vi "Protocol.RQST Wait on Response.vi"(0 "ref in":T3, 1 "Ignore Response":bool, 2 "Name":string, 5 "Source Address":u8=27, 7 "PGN":u32, 9 "DA":u8, 11 "error in (no error)":errorcluster, 12 "Processed Outgoing":refnum<queue>) -> (4 "element":T1 {"payload" format="%x"; "timestamp" format="%<%.7X\n%x>T"; "type" items=["CAN Data"=0, "CAN Remote"=1, "CAN Bus Error"=2, "CAN 2.0 Data"=8, "CAN FD Data"=16, "CAN FD+BRS Data"=24, "J1939 Data"=192, "Delay"=224, "Log Trigger"=225, "Start Trigger"=226]; "identifier" format="%x"}, 6 "timed out?":bool, 8 "Global Request?":bool, 15 "error out":errorcluster)   [LabVIEW 2019, in "J1939 Addon Engine.lvlib"]
uses:
  J1939 Addon Engine.lvlib
  Types/Protocol.RQST Lookup Table Reference.ctl
  <vilib>/xnet/xnet.llb/XNET Frame CAN.ctl
  <vilib>/xnet/xnet.llb/XNET Frame Type CAN.ctl
  Support Libraries/J1939 Utilities/Types/CAN Outgoing Message Cluster.ctl
  Types/Protocol.RQST Lookup Table Action.ctl
  Types/Protocol.RQST Lookup Table Cluster.ctl
  Support Libraries/J1939 Utilities/SubVIs/Request.vi
  Support Libraries/J1939 Utilities/Common Conversions.vi
  Support Libraries/J1939 Utilities/SubVIs/Convert J1939 ID to CAN Arb ID.vi
  Protocol.RQST Lookup Table.vi
  Support Libraries/J1939 Utilities/J1939 Utilities.lvlib
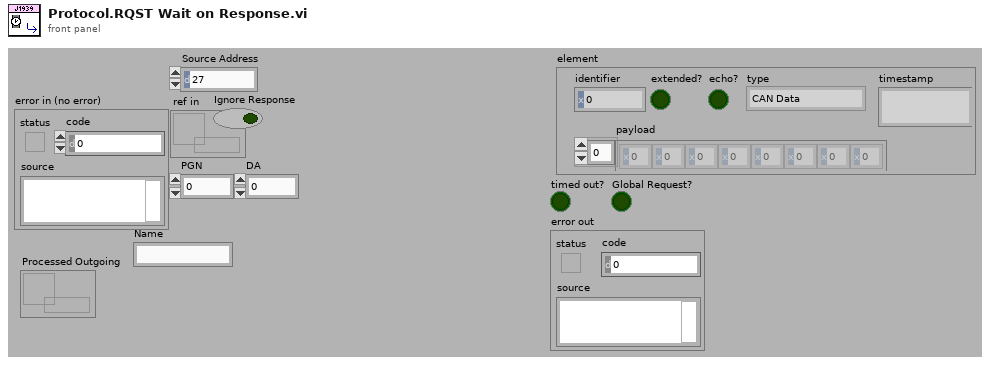
[diagram p1: front panel]
types:
  T1 = typedef "XNET Frame CAN.ctl" = cluster{"timestamp":timestamp, "payload":u8[], "identifier":u32, "type":T2, "extended?":bool, "echo?":bool}
  T2 = typedef "XNET Frame Type CAN.ctl" = u8
  T3 = typedef "J1939 Addon Engine.lvlib/Protocol.RQST Lookup Table Reference.ctl" = refnum<data-value>
  T4 = typedef "J1939 Utilities.lvlib/CAN Outgoing Message Cluster.ctl" = cluster{"Identifier":u32, "Data":u8[]}
  T5 = typedef "J1939 Addon Engine.lvlib/Protocol.RQST Lookup Table Action.ctl" = enum16{"Initialize", "Add", "Get", "Remove", "Get Active Requests"}
  T6 = typedef "J1939 Addon Engine.lvlib/Protocol.RQST Lookup Table Cluster.ctl" = cluster{"Response Q":refnum<queue>, "Request PGN":u32}
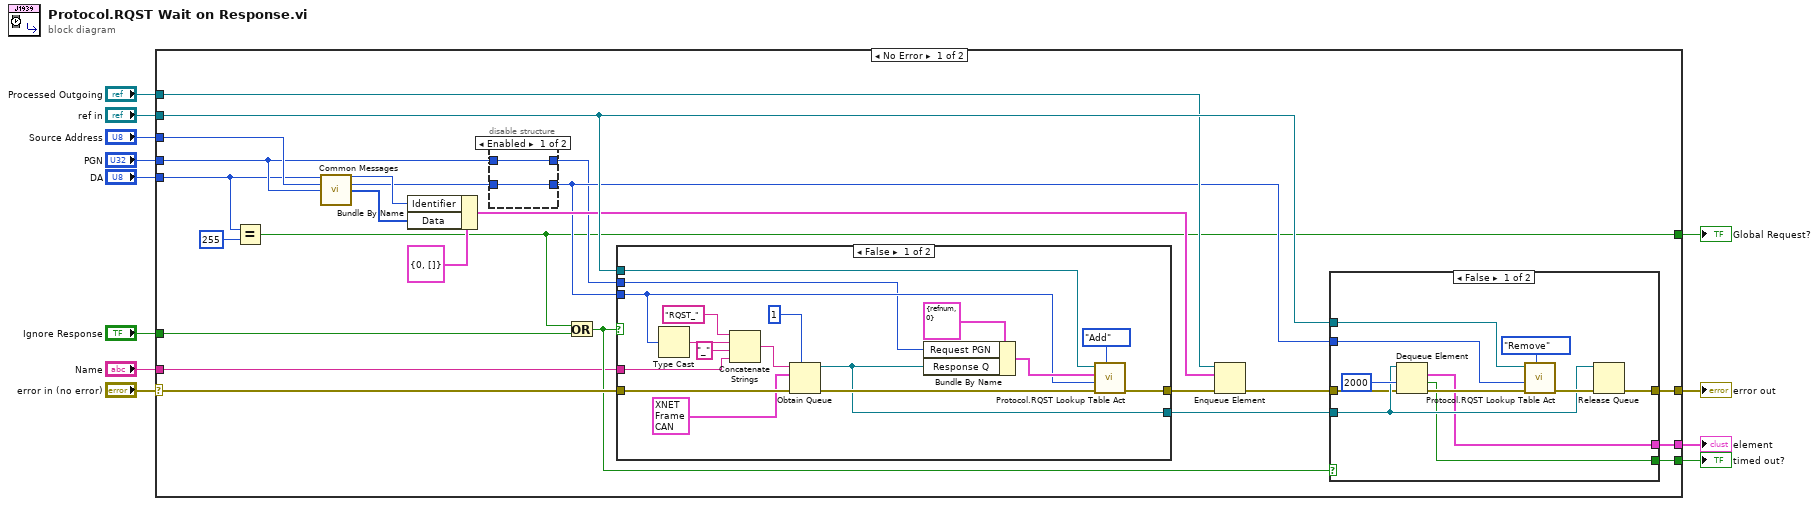
[diagram p0: block diagram]
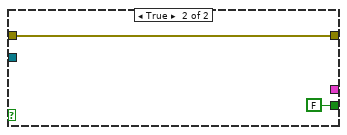
[diagram p2: hidden frame]
diagram:
  n1 = case shown="No Error" "error in (no error)" {
    selector: "error in (no error)" -> [w36 w71]
    tunnel: "Source Address" -> [w20 _]
    tunnel: "ref in" -> [w35 _]
    tunnel: [w33 w71] -> w8
    tunnel: [w32 _] -> w10
    tunnel: [w31 _] -> w9
    tunnel: "Processed Outgoing" -> [w28 _]
    tunnel: "PGN" -> [w19 _]
    tunnel: "DA" -> [w18 _]
    tunnel: [w14 _] -> w3
    tunnel: "Ignore Response" -> [w16 _]
    tunnel: "Name" -> [w13 _]
    frame No Error {
      n2 = Equal?(x=w18, y=u8 255) -> (x = y?=w14:bool)
      n3 = call-poly "Common Messages.vi"("Destination Address"=w18, "Source Address"=w20, "PGN"=w19) -> ("Arb ID"=w25:u32, "Expected Return Arb ID"=w23:u32, "Data"=w26:u8[])  [unwired: 10 in]
      n4 = Bundle By Name(cluster=T4 {"Identifier"=0, "Data"=[]} ("element"), "Identifier"=w25, "Data"=w26) -> (w24:T4)
      n5 = disable-structure shown="Enabled" {
        disable-tunnel: [w69 w70] -> w22
        disable-tunnel: w23 -> [w69 _]
        disable-tunnel: w19 -> [w68 w70]
        disable-tunnel: [w68 w70] -> w21
        frame Enabled {
        }
        frame Disabled {
        }
      }
      n6 = Or(x=w14, y=w16) -> (x .or. y?=w15:bool)
      n7 = case shown="False" w15 {
        tunnel: w36 -> [w65 w67]
        tunnel: w35 -> [w60 _]
        tunnel: [w59 _] -> w34
        tunnel: [w58 w67] -> w30
        tunnel: w22 -> [w52 _]
        tunnel: w21 -> [w51 _]
        tunnel: w13 -> [w53 _]
        frame False {
          n8 = Type Cast(x=w52) -> (*(type *) &x=w57:string)  [unwired: 1 in]
          n9 = Concatenate Strings("RQST_" ("string"), w57, "_" ("string"), w53) -> (w56:string)
          n10 = Obtain Queue(max queue size (-1, unlimited)=1, name (unnamed)=w56, element data type=T1 {"timestamp"=timestamp(0 s since 1904-01-01), "payload"=[], "identifier"=0, "type"=0, "extended?"=FALSE, "echo?"=FALSE} ("CAN frame"), error in (no error)=w65) -> (queue out=w59:refnum<queue>, error out=w64:errorcluster)  [unwired: 1 in, 1 out]
          n11 = Bundle By Name(cluster=T6 {"Response Q"=refnum, "Request PGN"=0} ("Data"), "Request PGN"=w51, "Response Q"=w59) -> (w61:T6)
          n12 = call "Protocol.RQST Lookup Table Act.vi"("Action"=Protocol.RQST_Lookup_Table_Action."Add", "error in (no error)"=w64, "ID"=w52, "Data"=w61, "Rqst LUT"=w60) -> ("error out"=w58:errorcluster)  [unwired: 2 in, 4 out]
        }
        frame True {
        }
      }
      n13 = Enqueue Element(queue=w28, element=w24, error in (no error)=w30) -> (error out=w29:errorcluster)  [unwired: 1 in, 2 out]
      n14 = case shown="False" w15 {
        tunnel: w35 -> [w45 _]
        tunnel: w34 -> [w43 _]
        tunnel: [w42 w49] -> w33
        tunnel: [w41 _] -> w32
        tunnel: [w40 FALSE ("timed out?")] -> w31
        tunnel: w29 -> [w39 w49]
        tunnel: w22 -> [w38 _]
        frame False {
          n15 = Dequeue Element(queue=w43, timeout in ms (-1)=2000, error in (no error)=w39) -> (element=w41:T1, timed out?=w40:bool, error out=w46:errorcluster)  [unwired: 1 out]
          n16 = call "Protocol.RQST Lookup Table Act.vi"("Action"=Protocol.RQST_Lookup_Table_Action."Remove", "error in (no error)"=w46, "ID"=w38, "Rqst LUT"=w45) -> ("error out"=w44:errorcluster)  [unwired: 3 in, 4 out]
          n17 = Release Queue(queue=w43, error in (no error)=w44) -> (error out=w42:errorcluster)  [unwired: 1 in, 2 out]
        }
        frame True {
        }
      }
    }
    frame Error {
    }
  }
  "element" <- w10
  "timed out?" <- w9
  "error out" <- w8
  "Global Request?" <- w3
